vi "Handle Error.vi"(8 "error in (no error)":errorcluster, 11 "HIJ Vision File Viewer App in":refnum<class "HIJ Vision File Viewer App.lvclass">) -> (0 "error out":errorcluster, 2 "stop actor?":bool=TRUE, 3 "HIJ Vision File Viewer App out":refnum<class "HIJ Vision File Viewer App.lvclass">)   [LabVIEW 2014, in "HIJ Vision File Viewer App.lvlib" / "HIJ Vision File Viewer App.lvclass"]
doc: "(<B>Filename</B>: Actor Framework.lvlib:Actor.lvclass:Handle Error.vi)\n\nDefines how the actor handles an error that occurred while processing a message. By default, this method does nothing except stop the actor."
uses:
  HIJ Vision File Viewer App.lvclass
  HIJ Vision Application/HIJ Vision Application/HIJ Vision Application.lvclass
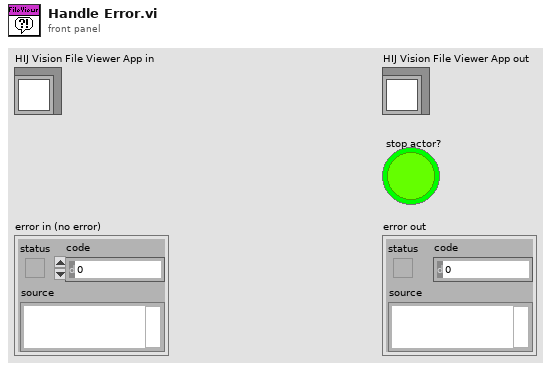
[diagram p1: front panel]
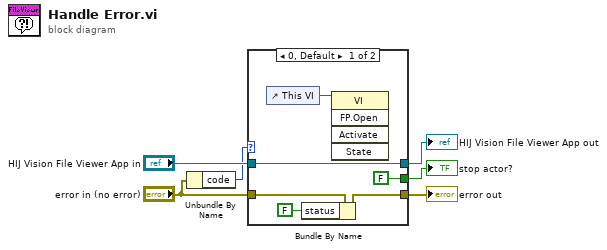
[diagram p0: block diagram]
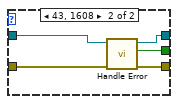
[diagram p2: hidden frame]
diagram:
  n1 = Unbundle By Name("error in (no error)") -> ("code"=w1:i32)
  n2 = case shown="0, Default" w1 {
    tunnel: [w8 w17] -> w6
    tunnel: [FALSE ("stop actor?") w16] -> w5
    tunnel: [w12 w15] -> w4
    tunnel: "HIJ Vision File Viewer App in" -> [w12 w14]
    tunnel: "error in (no error)" -> [w11 w13]
    frame 0, Default {
      n3 = control-ref of="This VI"() -> (w9:refnum<vi>)
      n4 = Bundle By Name(cluster=w11, "status"=FALSE) -> (w8:errorcluster)
      n5 = invoke class="VI" method="FP.Open"(reference=w9) -> ()  [unwired: 4 in, 5 out]
    }
    frame 43, 1608 {
      n6 = call-parent "Handle Error.vi"("error in (no error)"=w13, "Actor in"=w14) -> ("error out"=w17:errorcluster, "stop actor?"=w16:bool, "Actor out"=w15:refnum<class "HIJ Vision File Viewer App.lvclass">)  [unwired: 7 in]
    }
  }
  "HIJ Vision File Viewer App out" <- w4
  "error out" <- w6
  "stop actor?" <- w5
